vi "MICSD Get Attenuator.vi"(8 "error in (no error)":errorcluster, 11 "VISA Resource Name":refnum<visa-resource-name>) -> (0 "error out":errorcluster, 2 "Attenuation":u8, 3 "dup VISA Resource Name":refnum<visa-resource-name>)   [LabVIEW 2020]
uses:
  <vilib>/Instr/_visa.llb/VISA Configure Serial Port (Instr).vi
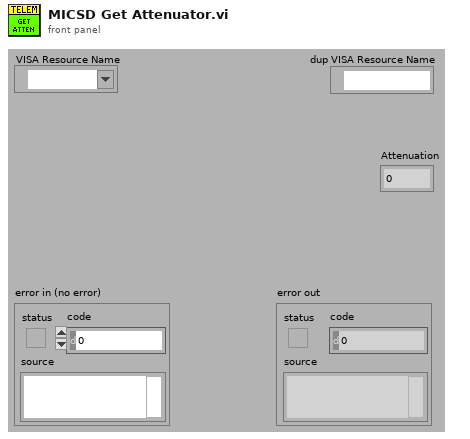
[diagram p1: front panel]
types:
  T1 = cluster{"Command Token":u8, "Length":u16, "Pack Data":u8[]}
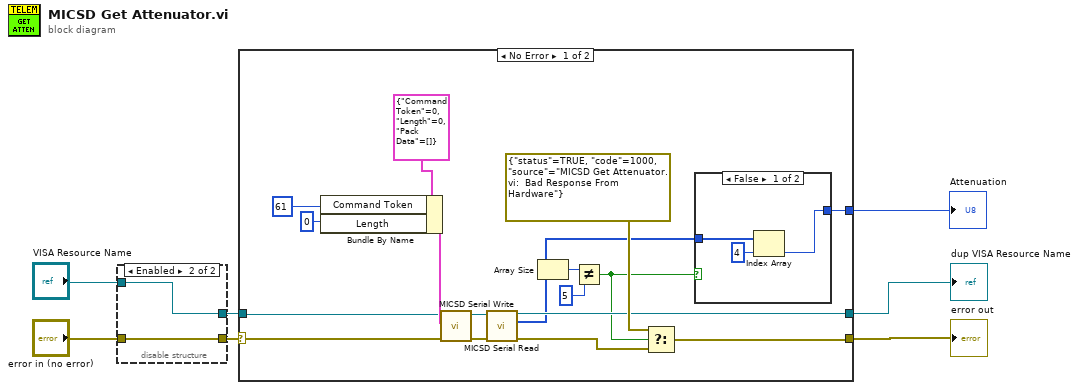
[diagram p0: block diagram]
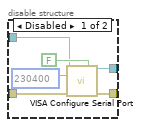
[diagram p2: hidden frame]
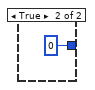
[diagram p3: hidden frame]
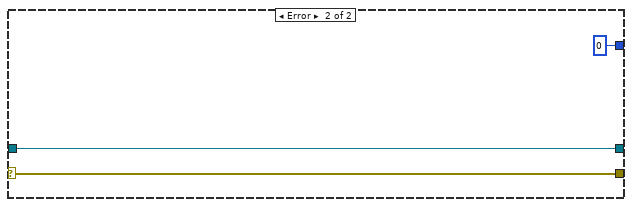
[diagram p4: hidden frame]
diagram:
  n1 = disable-structure shown="Enabled" {
    disable-tunnel: [w11 w14] -> w6
    disable-tunnel: "error in (no error)" -> [w10 w14]
    disable-tunnel: "VISA Resource Name" -> [w9 w15]
    disable-tunnel: [w8 w15] -> w3
    frame Disabled {
      n2 = call-poly "VISA Configure Serial Port"("VISA resource name"=w9, "Enable Termination\nChar (T)"=FALSE ("Enable Termination\nChar (T)"), "baud rate (9600)"=u32 230400, "error in (no error)"=w10) -> ("VISA resource name out"=w8:refnum<visa-resource-name>, "error out"=w11:errorcluster)  [unwired: 10 in]
    }
    frame Enabled {
    }
  }
  n3 = case shown="No Error" w6 {
    selector: w6 -> [w30 w39]
    tunnel: [w19 w39] -> w1
    tunnel: w3 -> [w29 w38]
    tunnel: [w21 w38] -> w7
    tunnel: [w17 u8 0 ("Attenuation")] -> w2
    frame No Error {
      n4 = Bundle By Name(cluster=T1 {"Command Token"=0, "Length"=0, "Pack Data"=[]} ("Write Data"), "Command Token"=u16 61 ("Length"), "Length"=u16 0) -> (w32:T1)
      n5 = call "MICSD Serial Write.vi"("error in (no error)"=w30, "Write Data"=w32, "VISA Resource Name"=w29) -> ("error out"=w26:errorcluster, "DUP Visa Resource Name"=w27:refnum<visa-resource-name>)  [unwired: 7 in]
      n6 = call "MICSD Serial Read.vi"("error in (no error)"=w26, "VISA Resource Name"=w27) -> ("error out"=w20:errorcluster, "Read Data"=w16:u8[], "DUP Visa Resource Name"=w21:refnum<visa-resource-name>)  [unwired: 7 in]
      n7 = Array Size(array=w16) -> (size(s)=w23:i32)
      n8 = Not Equal?(x=w23, y=5) -> (x != y?=w18:bool)
      n9 = Select(t=errorcluster {"status"=TRUE, "code"=1000, "source"="MICSD Get Attenuator.vi:  Bad Response From Hardware"} ("error IO"), s=w18, f=w20) -> (s? t:f=w19:errorcluster)
      n10 = case shown="False" w18 {
        tunnel: [w35 u8 0 ("Attenuation")] -> w17
        tunnel: w16 -> [w34 _]
        frame False {
          n11 = Index Array(array=w34, index=4) -> (element=w35:u8)
        }
        frame True {
        }
      }
    }
    frame Error {
    }
  }
  "dup VISA Resource Name" <- w7
  "error out" <- w1
  "Attenuation" <- w2
